vi "PNS Stoerungen Dynamisch.vi"(10 "Störmeldetexte":string, 11 "Nummer":i32) -> (3 "String":string)   [LabVIEW 2020, in "Stoerungen.lvlib"]
uses:
  Stoerungen.lvlib
  PNS/Aktionen FGV Loopkennung.ctl
  PNS/PNS.lvlib
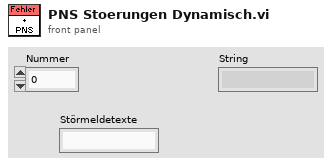
[diagram p1: front panel]
types:
  T1 = typedef "PNS.lvlib/Aktionen FGV Loopkennung.ctl" = enum16{"lesen", "schreiben"}
  T2 = typedef "PNS.lvlib/PNS Geraetekennung.ctl" = cluster{"Loops":string[], "Gerätetype":string, "Loopkennung":u16[], "Seriennummer":string, "Geraetekennung":u16, "SoftWare Version":string, "LP Kennung":u16}
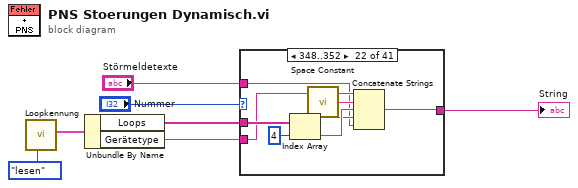
[diagram p0: block diagram]
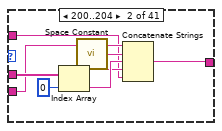
[diagram p3: hidden frame]
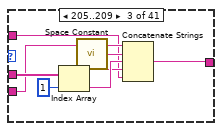
[diagram p4: hidden frame]
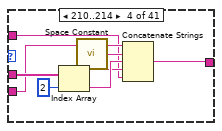
[diagram p5: hidden frame]
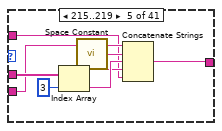
[diagram p6: hidden frame]
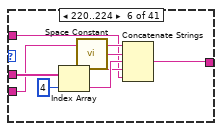
[diagram p7: hidden frame]
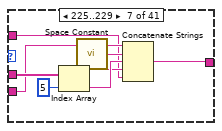
[diagram p8: hidden frame]
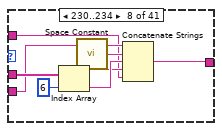
[diagram p9: hidden frame]
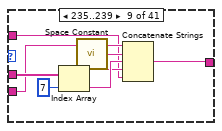
[diagram p10: hidden frame]
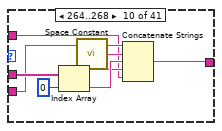
[diagram p11: hidden frame]
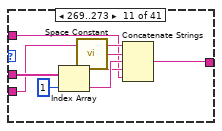
[diagram p12: hidden frame]
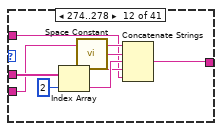
[diagram p13: hidden frame]
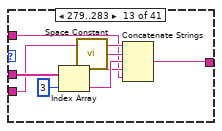
[diagram p14: hidden frame]
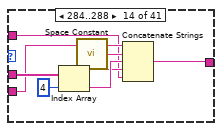
[diagram p15: hidden frame]
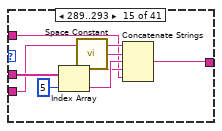
[diagram p16: hidden frame]
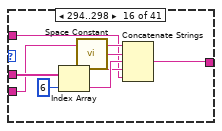
[diagram p17: hidden frame]
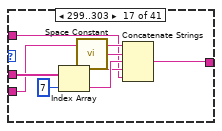
[diagram p18: hidden frame]
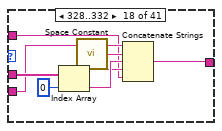
[diagram p19: hidden frame]
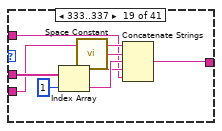
[diagram p20: hidden frame]
diagram:
  n1 = call "Loopkennung.vi"("Aktion"=Aktionen_FGV_Loopkennung."lesen") -> ("LoopGeraetekennung"=w5:T2)  [unwired: 9 in, 1 out]
  n2 = Unbundle By Name(w5) -> ("Loops"=w2:string[], "Gerätetype"=w1:string)
  n3 = case shown="348..352" "Nummer" {
    tunnel: "Störmeldetexte" -> [w8 w10 w17 w24 w31 w38 w45 w52 w59 w66 w73 w80 w87 w94 w101 w108 w115 w122 w129 w136 w143 w150 w157 w164 w171 w178 w185 w192 w199 w206 w213 w220 w227 w234 w241 w248 w255 w262 w269 w276 w283]
    tunnel: [w8 w9 w16 w23 w30 w37 w44 w51 w58 w65 w72 w79 w86 w93 w100 w107 w114 w121 w128 w135 w142 w149 w156 w163 w170 w177 w184 w191 w198 w205 w212 w219 w226 w233 w240 w247 w254 w261 w268 w275 w282] -> w7
    tunnel: w2 -> [_ w15 w22 w29 w36 w43 w50 w57 w64 w71 w78 w85 w92 w99 w106 w113 w120 w127 w134 w141 w148 w155 w162 w169 w176 w183 w190 w197 w204 w211 w218 w225 w232 w239 w246 w253 w260 w267 w274 w281 w288]
    tunnel: w1 -> [_ w13 w20 w27 w34 w41 w48 w55 w62 w69 w76 w83 w90 w97 w104 w111 w118 w125 w132 w139 w146 w153 w160 w167 w174 w181 w188 w195 w202 w209 w216 w223 w230 w237 w244 w251 w258 w265 w272 w279 w286]
    frame 0, Default {
    }
    frame 200..204 {
      n4 = Index Array(array=w15, index=0 ("Index")) -> (element=w12:string)
      n5 = call <vilib>:"Space Constant.vi"() -> ("String"=w11:string)
      n6 = Concatenate Strings(w13, w11, w12, w11, w10) -> (w9:string)
    }
    frame 205..209 {
      n7 = Index Array(array=w22, index=1 ("Index")) -> (element=w19:string)
      n8 = call <vilib>:"Space Constant.vi"() -> ("String"=w18:string)
      n9 = Concatenate Strings(w20, w18, w19, w18, w17) -> (w16:string)
    }
    frame 210..214 {
      n10 = Index Array(array=w29, index=2 ("Index")) -> (element=w26:string)
      n11 = call <vilib>:"Space Constant.vi"() -> ("String"=w25:string)
      n12 = Concatenate Strings(w27, w25, w26, w25, w24) -> (w23:string)
    }
    frame 215..219 {
      n13 = Index Array(array=w36, index=3 ("Index")) -> (element=w33:string)
      n14 = call <vilib>:"Space Constant.vi"() -> ("String"=w32:string)
      n15 = Concatenate Strings(w34, w32, w33, w32, w31) -> (w30:string)
    }
    frame 220..224 {
      n16 = Index Array(array=w43, index=4 ("Index")) -> (element=w40:string)
      n17 = call <vilib>:"Space Constant.vi"() -> ("String"=w39:string)
      n18 = Concatenate Strings(w41, w39, w40, w39, w38) -> (w37:string)
    }
    frame 225..229 {
      n19 = Index Array(array=w50, index=5 ("Index")) -> (element=w47:string)
      n20 = call <vilib>:"Space Constant.vi"() -> ("String"=w46:string)
      n21 = Concatenate Strings(w48, w46, w47, w46, w45) -> (w44:string)
    }
    frame 230..234 {
      n22 = Index Array(array=w57, index=6 ("Index")) -> (element=w54:string)
      n23 = call <vilib>:"Space Constant.vi"() -> ("String"=w53:string)
      n24 = Concatenate Strings(w55, w53, w54, w53, w52) -> (w51:string)
    }
    frame 235..239 {
      n25 = Index Array(array=w64, index=7 ("Index")) -> (element=w61:string)
      n26 = call <vilib>:"Space Constant.vi"() -> ("String"=w60:string)
      n27 = Concatenate Strings(w62, w60, w61, w60, w59) -> (w58:string)
    }
    frame 264..268 {
      n28 = Index Array(array=w71, index=0 ("Index")) -> (element=w68:string)
      n29 = call <vilib>:"Space Constant.vi"() -> ("String"=w67:string)
      n30 = Concatenate Strings(w69, w67, w68, w67, w66) -> (w65:string)
    }
    frame 269..273 {
      n31 = Index Array(array=w78, index=1 ("Index")) -> (element=w75:string)
      n32 = call <vilib>:"Space Constant.vi"() -> ("String"=w74:string)
      n33 = Concatenate Strings(w76, w74, w75, w74, w73) -> (w72:string)
    }
    frame 274..278 {
      n34 = Index Array(array=w85, index=2 ("Index")) -> (element=w82:string)
      n35 = call <vilib>:"Space Constant.vi"() -> ("String"=w81:string)
      n36 = Concatenate Strings(w83, w81, w82, w81, w80) -> (w79:string)
    }
    frame 279..283 {
      n37 = Index Array(array=w92, index=3 ("Index")) -> (element=w89:string)
      n38 = call <vilib>:"Space Constant.vi"() -> ("String"=w88:string)
      n39 = Concatenate Strings(w90, w88, w89, w88, w87) -> (w86:string)
    }
    frame 284..288 {
      n40 = Index Array(array=w99, index=4 ("Index")) -> (element=w96:string)
      n41 = call <vilib>:"Space Constant.vi"() -> ("String"=w95:string)
      n42 = Concatenate Strings(w97, w95, w96, w95, w94) -> (w93:string)
    }
    frame 289..293 {
      n43 = Index Array(array=w106, index=5 ("Index")) -> (element=w103:string)
      n44 = call <vilib>:"Space Constant.vi"() -> ("String"=w102:string)
      n45 = Concatenate Strings(w104, w102, w103, w102, w101) -> (w100:string)
    }
    frame 294..298 {
      n46 = Index Array(array=w113, index=6 ("Index")) -> (element=w110:string)
      n47 = call <vilib>:"Space Constant.vi"() -> ("String"=w109:string)
      n48 = Concatenate Strings(w111, w109, w110, w109, w108) -> (w107:string)
    }
    frame 299..303 {
      n49 = Index Array(array=w120, index=7 ("Index")) -> (element=w117:string)
      n50 = call <vilib>:"Space Constant.vi"() -> ("String"=w116:string)
      n51 = Concatenate Strings(w118, w116, w117, w116, w115) -> (w114:string)
    }
    frame 328..332 {
      n52 = Index Array(array=w127, index=0 ("Index")) -> (element=w124:string)
      n53 = call <vilib>:"Space Constant.vi"() -> ("String"=w123:string)
      n54 = Concatenate Strings(w125, w123, w124, w123, w122) -> (w121:string)
    }
    frame 333..337 {
      n55 = Index Array(array=w134, index=1 ("Index")) -> (element=w131:string)
      n56 = call <vilib>:"Space Constant.vi"() -> ("String"=w130:string)
      n57 = Concatenate Strings(w132, w130, w131, w130, w129) -> (w128:string)
    }
    frame 338..342 {
      n58 = Index Array(array=w141, index=2 ("Index")) -> (element=w138:string)
      n59 = call <vilib>:"Space Constant.vi"() -> ("String"=w137:string)
      n60 = Concatenate Strings(w139, w137, w138, w137, w136) -> (w135:string)
    }
    frame 343..347 {
      n61 = Index Array(array=w148, index=3 ("Index")) -> (element=w145:string)
      n62 = call <vilib>:"Space Constant.vi"() -> ("String"=w144:string)
      n63 = Concatenate Strings(w146, w144, w145, w144, w143) -> (w142:string)
    }
    frame 348..352 {
      n64 = Index Array(array=w155, index=4 ("Index")) -> (element=w152:string)
      n65 = call <vilib>:"Space Constant.vi"() -> ("String"=w151:string)
      n66 = Concatenate Strings(w153, w151, w152, w151, w150) -> (w149:string)
    }
    frame 353..357 {
      n67 = Index Array(array=w162, index=5 ("Index")) -> (element=w159:string)
      n68 = call <vilib>:"Space Constant.vi"() -> ("String"=w158:string)
      n69 = Concatenate Strings(w160, w158, w159, w158, w157) -> (w156:string)
    }
    frame 358..362 {
      n70 = Index Array(array=w169, index=6 ("Index")) -> (element=w166:string)
      n71 = call <vilib>:"Space Constant.vi"() -> ("String"=w165:string)
      n72 = Concatenate Strings(w167, w165, w166, w165, w164) -> (w163:string)
    }
    frame 363..367 {
      n73 = Index Array(array=w176, index=7 ("Index")) -> (element=w173:string)
      n74 = call <vilib>:"Space Constant.vi"() -> ("String"=w172:string)
      n75 = Concatenate Strings(w174, w172, w173, w172, w171) -> (w170:string)
    }
    frame 392..396 {
      n76 = Index Array(array=w183, index=0 ("Index")) -> (element=w180:string)
      n77 = call <vilib>:"Space Constant.vi"() -> ("String"=w179:string)
      n78 = Concatenate Strings(w181, w179, w180, w179, w178) -> (w177:string)
    }
    frame 397..401 {
      n79 = Index Array(array=w190, index=1 ("Index")) -> (element=w187:string)
      n80 = call <vilib>:"Space Constant.vi"() -> ("String"=w186:string)
      n81 = Concatenate Strings(w188, w186, w187, w186, w185) -> (w184:string)
    }
    frame 402..406 {
      n82 = Index Array(array=w197, index=2 ("Index")) -> (element=w194:string)
      n83 = call <vilib>:"Space Constant.vi"() -> ("String"=w193:string)
      n84 = Concatenate Strings(w195, w193, w194, w193, w192) -> (w191:string)
    }
    frame 407..411 {
      n85 = Index Array(array=w204, index=3 ("Index")) -> (element=w201:string)
      n86 = call <vilib>:"Space Constant.vi"() -> ("String"=w200:string)
      n87 = Concatenate Strings(w202, w200, w201, w200, w199) -> (w198:string)
    }
    frame 412..416 {
      n88 = Index Array(array=w211, index=4 ("Index")) -> (element=w208:string)
      n89 = call <vilib>:"Space Constant.vi"() -> ("String"=w207:string)
      n90 = Concatenate Strings(w209, w207, w208, w207, w206) -> (w205:string)
    }
    frame 417..421 {
      n91 = Index Array(array=w218, index=5 ("Index")) -> (element=w215:string)
      n92 = call <vilib>:"Space Constant.vi"() -> ("String"=w214:string)
      n93 = Concatenate Strings(w216, w214, w215, w214, w213) -> (w212:string)
    }
    frame 422..426 {
      n94 = Index Array(array=w225, index=6 ("Index")) -> (element=w222:string)
      n95 = call <vilib>:"Space Constant.vi"() -> ("String"=w221:string)
      n96 = Concatenate Strings(w223, w221, w222, w221, w220) -> (w219:string)
    }
    frame 427..431 {
      n97 = Index Array(array=w232, index=7 ("Index")) -> (element=w229:string)
      n98 = call <vilib>:"Space Constant.vi"() -> ("String"=w228:string)
      n99 = Concatenate Strings(w230, w228, w229, w228, w227) -> (w226:string)
    }
    frame 456..460 {
      n100 = Index Array(array=w239, index=0 ("Index")) -> (element=w236:string)
      n101 = call <vilib>:"Space Constant.vi"() -> ("String"=w235:string)
      n102 = Concatenate Strings(w237, w235, w236, w235, w234) -> (w233:string)
    }
    frame 461..465 {
      n103 = Index Array(array=w246, index=1 ("Index")) -> (element=w243:string)
      n104 = call <vilib>:"Space Constant.vi"() -> ("String"=w242:string)
      n105 = Concatenate Strings(w244, w242, w243, w242, w241) -> (w240:string)
    }
    frame 466..470 {
      n106 = Index Array(array=w253, index=2 ("Index")) -> (element=w250:string)
      n107 = call <vilib>:"Space Constant.vi"() -> ("String"=w249:string)
      n108 = Concatenate Strings(w251, w249, w250, w249, w248) -> (w247:string)
    }
    frame 471..475 {
      n109 = Index Array(array=w260, index=3 ("Index")) -> (element=w257:string)
      n110 = call <vilib>:"Space Constant.vi"() -> ("String"=w256:string)
      n111 = Concatenate Strings(w258, w256, w257, w256, w255) -> (w254:string)
    }
    frame 476..480 {
      n112 = Index Array(array=w267, index=4 ("Index")) -> (element=w264:string)
      n113 = call <vilib>:"Space Constant.vi"() -> ("String"=w263:string)
      n114 = Concatenate Strings(w265, w263, w264, w263, w262) -> (w261:string)
    }
    frame 481..485 {
      n115 = Index Array(array=w274, index=5 ("Index")) -> (element=w271:string)
      n116 = call <vilib>:"Space Constant.vi"() -> ("String"=w270:string)
      n117 = Concatenate Strings(w272, w270, w271, w270, w269) -> (w268:string)
    }
    frame 486..490 {
      n118 = Index Array(array=w281, index=6 ("Index")) -> (element=w278:string)
      n119 = call <vilib>:"Space Constant.vi"() -> ("String"=w277:string)
      n120 = Concatenate Strings(w279, w277, w278, w277, w276) -> (w275:string)
    }
    frame 491..495 {
      n121 = Index Array(array=w288, index=7 ("Index")) -> (element=w285:string)
      n122 = call <vilib>:"Space Constant.vi"() -> ("String"=w284:string)
      n123 = Concatenate Strings(w286, w284, w285, w284, w283) -> (w282:string)
    }
  }
  "String" <- w7
